vi "oa_Check XY Output Availability.vi"(8 "error in (no error)":errorcluster, 9 "reached end?":bool, 10 "XY signal":cluster{"X":dbl[], "Y":dbl[]} {"X" format="%.2f"; "Y" format="%.2f"}, 11 "x-axis selection":u16(ring)=2 items=["Time", "Revolution", "RPM"]) -> (0 "error out":errorcluster)   [LabVIEW 2017, in "SoundVib_OAUtility.lvlib"]
uses:
  <vilib>/addons/Sound and Vibration/Order Analysis/Utility/SoundVib_OAUtility.lvlib
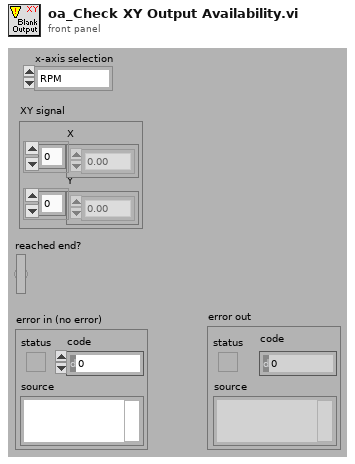
[diagram p1: front panel]
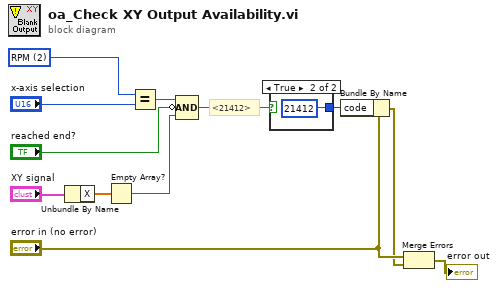
[diagram p0: block diagram]
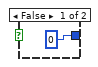
[diagram p2: hidden frame]
diagram:
  w1 = u16 2 items=["Time", "Revolution", "RPM"] ("x-axis selection")
  # "<21412>"
  n1 = Unbundle By Name("XY signal") -> ("X"=w4:dbl[])
  n2 = Empty Array?(array=w4) -> (empty?=w3:bool)
  n3 = Equal?(x=w1, y="x-axis selection") -> (x = y?=w8:bool)
  n4 = Compound Arithmetic op=AND(w8, invert "reached end?", w3) -> (w6:bool)
  n5 = case shown="True" w6 {
    tunnel: [0 ("code") 21412 ("code")] -> w10
    frame False {
    }
    frame True {
    }
  }
  n6 = Bundle By Name(cluster="error in (no error)", "code"=w10) -> (w9:errorcluster)
  n7 = Merge Errors("error in (no error)", w9) -> (→"error out":errorcluster)
